vi "Configure Channel Expand and Offset.vi"(5 "Manual Offset (0)":dbl, 7 "Auto Offset (F: Disable)":bool, 8 "error in (no error)":errorcluster, 9 "Expand (0: x1)":u16(ring) items=["x1", "x10", "x100"], 10 "Offset/Expand Parameter (1: X)":u16(ring)=1 items=["X"=1, "Y"=2, "R"=3], 11 "VISA resource name":refnum<visa-resource-name>) -> (0 "error out":errorcluster, 3 "VISA resource name out":refnum<visa-resource-name>)   [LabVIEW 2012, in "Stanford Research 830.lvlib"]
doc: "Configures the expand and offset of the instrument's display via the formula:\nIf the parameter selected is X, then\n\nDisplay = (X/Sensitivity - Offset) x Expand\n\n<B>Note:</B>\n\nThe setting in this VI will affect the channel output and the channel display."
uses:
  Stanford Research 830.lvlib
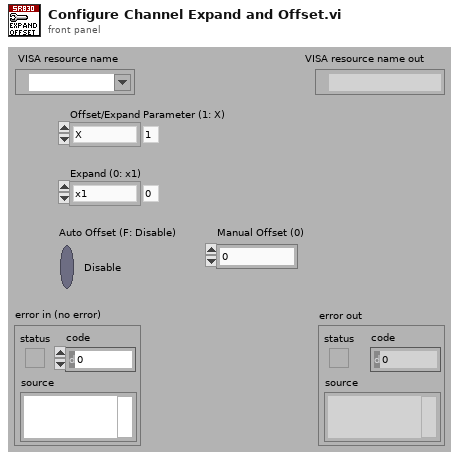
[diagram p1: front panel]
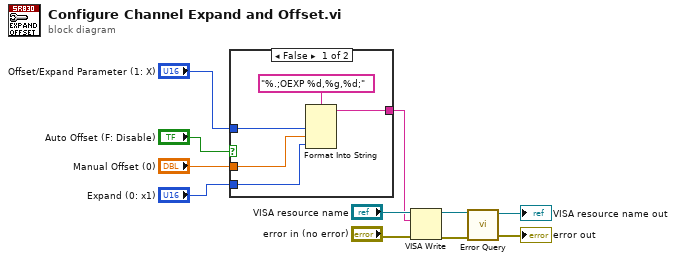
[diagram p0: block diagram]
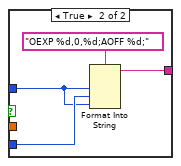
[diagram p2: hidden frame]
diagram:
  n1 = case shown="False" "Auto Offset (F: Disable)" {
    tunnel: "Expand (0: x1)" -> [w14 w18]
    tunnel: "Manual Offset (0)" -> [w15 _]
    tunnel: "Offset/Expand Parameter (1: X)" -> [w13 w17]
    tunnel: [w12 w19] -> w5
    frame False {
      n2 = Format Into String(format string="%.;OEXP %d,%g,%d;", w13, w15, w14) -> (resulting string=w12:string)  [unwired: 2 in, 1 out]
    }
    frame True {
      n3 = Format Into String(format string="OEXP %d,0,%d;AOFF %d;", w17, w18, w17) -> (resulting string=w19:string)  [unwired: 2 in, 1 out]
    }
  }
  n4 = VISA Write(VISA resource name="VISA resource name", write buffer=w5, error in (no error)="error in (no error)") -> (VISA resource name out=w2:refnum<visa-resource-name>, error out=w1:errorcluster)  [unwired: 1 out]
  n5 = call "Error Query.vi"("error in (no error)"=w1, "VISA resource name"=w2) -> ("error out"=→"error out":errorcluster, "VISA resource name out"=→"VISA resource name out":refnum<visa-resource-name>)  [unwired: 7 in, 1 out]
